vi "Export Dialog.vi"(8 "error in (no error)":errorcluster, 11 "Item Ref in":T1 format="%.0x") -> (0 "error out":errorcluster, 3 "Item Ref out":T1 format="%.0x")   [LabVIEW 2020, in "DSF System Explorer.lvlib"]
uses:
  DSF System Explorer.lvlib
  <vilib>/NI VeriStand/Custom Device API/Custom Device Item Ref.ctl
  Includes/DSF Core.lvlibp/Typedefs/DSF Engine Framework Configuration.ctl
  Includes/DSF Core.lvlibp/Typedefs/DSF Engine Plugin Configuration.ctl
  Includes/DSF Core.lvlibp/Typedefs/Core Plugin Configuration.ctl
  Includes/DSF Core.lvlibp/Typedefs/DSF Timing Info.ctl
  Includes/DSF Core.lvlibp/Typedefs/DSF Settings Info.ctl
  Includes/DSF Core.lvlibp/Typedefs/DSF Engine Plugin Thread Configuration.ctl
  Includes/DSF Core.lvlibp/Typedefs/Core Thread Configuration.ctl
  Includes/DSF Core.lvlibp/Typedefs/DSF Engine Transfer Group Configuration.ctl
  Includes/DSF Core.lvlibp/Typedefs/Core Group Configuration.ctl
  Includes/DSF Core.lvlibp/Typedefs/DSF Direction.ctl
  Includes/DSF Core.lvlibp/Typedefs/DSF Timeout Behavior.ctl
  Includes/DSF Core.lvlibp/Typedefs/DSF Engine Transfer Configuration.ctl
  Includes/DSF Core.lvlibp/Typedefs/Core Transfer Configuration.ctl
  Includes/DSF Core.lvlibp/Typedefs/DSF Engine Channel Configuration.ctl
  Includes/DSF Core.lvlibp/Typedefs/Core Channel Configuration.ctl
  Includes/DSF Core.lvlibp/Typedefs/DSF Data Type.ctl
  Includes/DSF Core.lvlibp
  Includes/DSF Core.lvlibp/Classes/Configuration/Core/Plugin/Plugin Configuration.lvclass
  Includes/DSF Core.lvlibp/Classes/Configuration/Core/Thread/Thread Configuration.lvclass
  Includes/DSF Core.lvlibp/Classes/Configuration/Core/Group/Group Configuration.lvclass
  Includes/DSF Core.lvlibp/Classes/Configuration/Core/Transfer/Transfer Configuration.lvclass
  Includes/DSF Core.lvlibp/Classes/Configuration/Core/Channel/Channel Configuration.lvclass
  Includes/DSF Core.lvlibp/Classes/Configuration Session/Configuration Session.lvclass
  Shared/DSF Shared.lvlib
  <vilib>/NI VeriStand/Custom Device API/Custom Device API.lvlib
panel:
  out "Duration":u32 format="%d ms"
  out "Version":string
  in  "Generate":bool
  in  "Save":bool
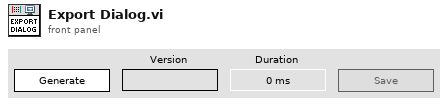
[diagram p1: front panel]
types:
  T1 = typedef "Custom Device API.lvlib/Custom Device Item Ref.ctl" = u64
  T2 = enum8{"Enabled", "Disabled", "Disabled and Grayed Out"}
  T3 = typedef "DSF Core.lvlibp/DSF Engine Framework Configuration.ctl" = cluster{"plugins":T4[]}
  T4 = typedef "DSF Core.lvlibp/DSF Engine Plugin Configuration.ctl" = cluster{"core":T5, "component settings":T7[], "threads":T8[]}
  T5 = typedef "DSF Core.lvlibp/Plugin Configuration.lvclass/Core Plugin Configuration.ctl" = cluster{"name":string, "components":string[], "cycle timing":T6}
  T6 = typedef "DSF Core.lvlibp/DSF Timing Info.ctl" = cluster{"priority":u64, "decimation":u64, "offset":u64}
  T7 = typedef "DSF Core.lvlibp/DSF Settings Info.ctl" = cluster{"component":string, "values":cluster{"key":string, "value":string}[]}
  T8 = typedef "DSF Core.lvlibp/DSF Engine Plugin Thread Configuration.ctl" = cluster{"core":T9, "component settings":T7[], "transfer groups":T10[]}
  T9 = typedef "DSF Core.lvlibp/Thread Configuration.lvclass/Core Thread Configuration.ctl" = cluster{"processor":i32, "priority offset":i16}
  T10 = typedef "DSF Core.lvlibp/DSF Engine Transfer Group Configuration.ctl" = cluster{"core":T11, "component settings":T7[], "transfers":T14[]}
  T11 = typedef "DSF Core.lvlibp/Group Configuration.lvclass/Core Group Configuration.ctl" = cluster{"name":string, "direction":T12, "cycle timing":T6, "timeout behavior":T13, "enable conversion":bool}
  T12 = typedef "DSF Core.lvlibp/DSF Direction.ctl" = enum8{"Tx", "Rx"}
  T13 = typedef "DSF Core.lvlibp/DSF Timeout Behavior.ctl" = enum8{"Increment Late Count", "Throw Error"}
  T14 = typedef "DSF Core.lvlibp/DSF Engine Transfer Configuration.ctl" = cluster{"core":T15, "component settings":T7[], "channels":T16[]}
  T15 = typedef "DSF Core.lvlibp/Transfer Configuration.lvclass/Core Transfer Configuration.ctl" = cluster{"name":string}
  T16 = typedef "DSF Core.lvlibp/DSF Engine Channel Configuration.ctl" = cluster{"core":T17, "component settings":T7[]}
  T17 = typedef "DSF Core.lvlibp/Channel Configuration.lvclass/Core Channel Configuration.ctl" = cluster{"name":string, "units":string, "engine data type":T18, "string data type":T18, "string offset":u64}
  T18 = typedef "DSF Core.lvlibp/DSF Data Type.ctl" = enum8{"Bool", "SGL", "DBL", "I8", "I16", "I32", "I64", "U8", "U16", "U32", "U64"}
  T19 = typedef "DSF Core.lvlibp/DSF Version Info.ctl" = cluster{"major":u32, "minor":u32, "fix":u32, "build":string}
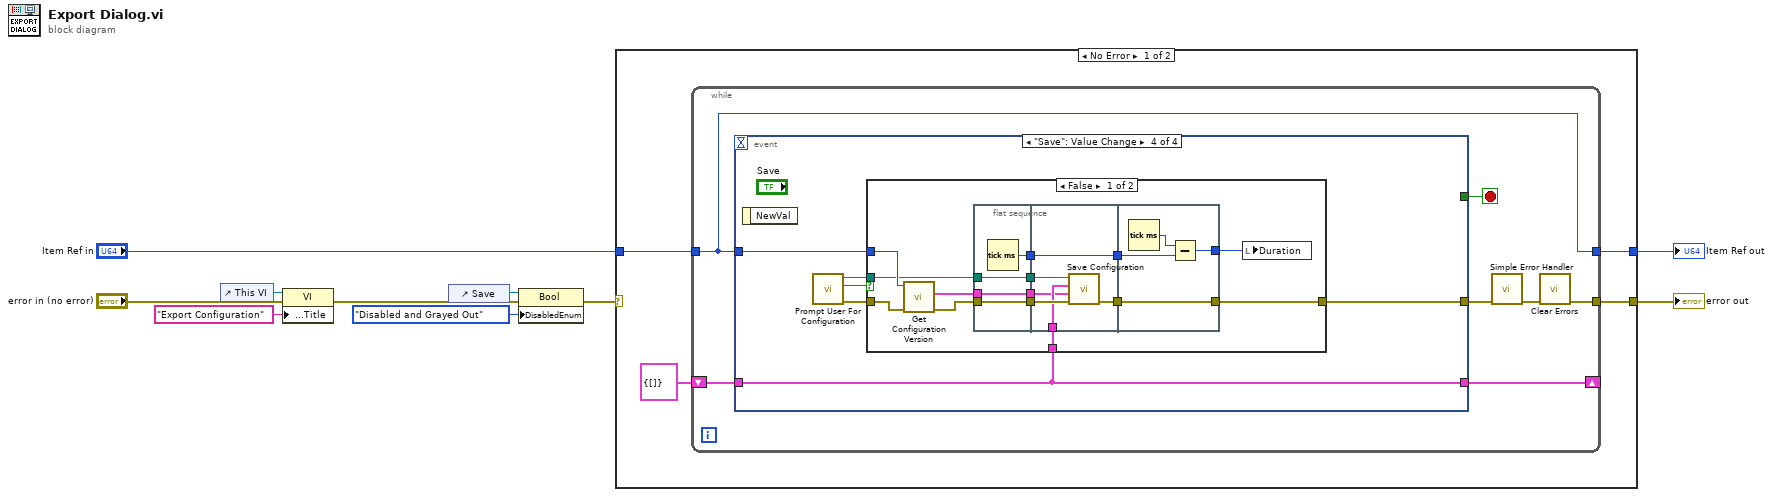
[diagram p0: block diagram]
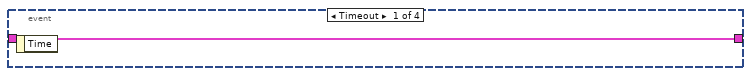
[diagram p2: hidden frame]
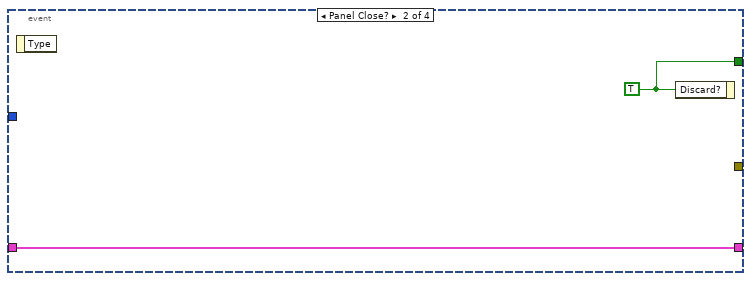
[diagram p3: hidden frame]
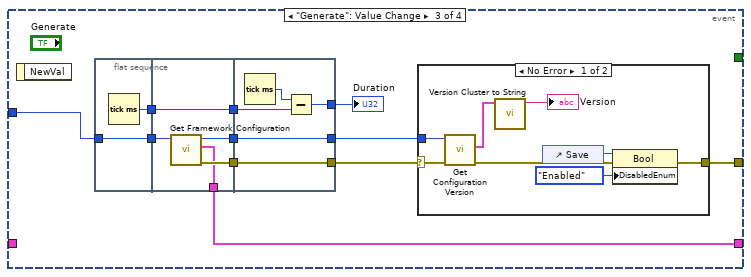
[diagram p4: hidden frame]
diagram:
  n1 = control-ref of="This VI"() -> (w7:refnum<vi>)
  n2 = property class="VI"(reference=w7, error in="error in (no error)", "Front Panel.Title"="Export Configuration" ("Front Panel Window:Title")) -> (error out=w2:errorcluster)  [unwired: 1 out]
  n3 = control-ref of="Save"() -> (w3:refnum<vi>)
  n4 = property class="Bool"(reference=w3, error in=w2, "DisabledEnum"=T2."Disabled and Grayed Out" ("Disabled")) -> (error out=w1:errorcluster)  [unwired: 1 out]
  n5 = case shown="No Error" w1 {
    selector: w1 -> [_ w92]
    tunnel: [w14 w92] -> w10
    tunnel: "Item Ref in" -> [w13 w93]
    tunnel: [w12 w93] -> w8
    frame No Error {
      n6 = while {
        tunnel: w13 -> [w15]
        tunnel: [w15] -> w12
        shift-right: [w17] -> _
        shift-left: T3 {"plugins"=[]} ("framework configuration") -> [w16]
        tunnel: [w20] -> w14
        stop <- w21 stop-if-true
        n7 = event shown="[3] \"Save\": Value Change" {
          selector: _ -> [_ _ _ _]
          dyn-events: _ -> [_ _ _ _]
          timeout: _ -> [_ _ _ _]
          tunnel: [_ w23 _ _] -> w21
          tunnel: [_ _ w30 w57] -> w19
          tunnel: w16 -> [w22 w24 _ w58]
          tunnel: [w22 w24 w29 w58] -> w17
          tunnel: w15 -> [_ _ w28 w59]
          event Timeout {
            n8 = event-data() -> ()  [unwired: 1 in, 1 out]
          }
          event Panel Close? {
            w23 = TRUE ("Discard?")
            n9 = event-data() -> ()  [unwired: 1 in, 1 out]
            n10 = event-data("Discard?"=w23) -> ()  [unwired: 1 in, 1 out]
          }
          event "Generate": Value Change {
            n11 = event-data() -> ()  [unwired: 1 in, 1 out]
            n12 = flat-sequence {
              tunnel: [w46] -> w35
              tunnel: w28 -> [w45]
              tunnel: [w45] -> w27
              tunnel: w35 -> [w51]
              tunnel: [w51] -> w34
              tunnel: [w50] -> w32
              tunnel: [w49] -> w29
              tunnel: w27 -> [w48]
              tunnel: [w47] -> w26
              tunnel: w34 -> [w56]
              tunnel: [w54] -> w33
              tunnel: w32 -> [w53]
              tunnel: [w53] -> w31
              tunnel: w26 -> [w52]
              tunnel: [w52] -> w25
              frame #0 {
                n13 = Tick Count (ms)() -> (millisecond timer value=w46:u32)
              }
              frame #1 {
                n14 = call "Get Framework Configuration.vi"("Item Ref in"=w48) -> ("error out"=w50:errorcluster, "framework configuration"=w49:T3, "Item Ref out"=w47:T1)  [unwired: 8 in]
              }
              frame #2 {
                n15 = Tick Count (ms)() -> (millisecond timer value=w55:u32)
                n16 = Subtract(x=w55, y=w56) -> (x-y=w54:u32)
              }
            }
            n17 = case shown="No Error" w31 {
              selector: w31 -> [w41 w44]
              tunnel: [w36 w44] -> w30
              tunnel: w25 -> [w40 _]
              frame No Error {
                n18 = call "Get Configuration Version.vi"("error in (no error)"=w41, "Item Ref in"=w40) -> ("error out"=w37:errorcluster, "version"=w38:T19)  [unwired: 7 in, 1 out]
                n19 = call "Version Cluster to String.vi"("version"=w38) -> ("version string"=→"Version":string)  [unwired: 9 in, 1 out]
                n20 = control-ref of="Save"() -> (w43:refnum<vi>)
                n21 = property class="Bool"(reference=w43, error in=w37, "DisabledEnum"=T2."Enabled" ("Disabled")) -> (error out=w36:errorcluster)  [unwired: 1 out]
              }
              frame Error {
              }
            }
            "Duration" <- w33
          }
          event "Save": Value Change {
            n22 = event-data() -> ()  [unwired: 1 in, 1 out]
            n23 = call "Prompt User For Configuration.vi"() -> ("error out"=w62:errorcluster, "cancelled"=w60:bool, "selected path"=w61:path)  [unwired: 9 in]
            n24 = case shown="False" w60 {
              tunnel: [w71 w91] -> w57
              tunnel: w62 -> [w69 w91]
              tunnel: w61 -> [w63 _]
              tunnel: w58 -> [w70 _]
              tunnel: w59 -> [w68 _]
              frame False {
                n25 = call "Get Configuration Version.vi"("error in (no error)"=w69, "Item Ref in"=w68) -> ("error out"=w67:errorcluster, "version"=w65:T19)  [unwired: 7 in, 1 out]
                n26 = flat-sequence {
                  tunnel: w67 -> [w80]
                  tunnel: [w80] -> w76
                  tunnel: [w79] -> w74
                  tunnel: w63 -> [w78]
                  tunnel: [w78] -> w66
                  tunnel: w65 -> [w77]
                  tunnel: [w77] -> w64
                  tunnel: w76 -> [w85]
                  tunnel: [w86] -> w75
                  tunnel: w74 -> [w84]
                  tunnel: [w84] -> w73
                  tunnel: w70 -> [w83]
                  tunnel: w66 -> [w82]
                  tunnel: w64 -> [w81]
                  tunnel: [w90] -> w71
                  tunnel: w75 -> [w90]
                  tunnel: w73 -> [w89]
                  tunnel: [w87] -> w72
                  frame #0 {
                    n27 = Tick Count (ms)() -> (millisecond timer value=w79:u32)
                  }
                  frame #1 {
                    n28 = call "Save Configuration.vi"("error in (no error)"=w85, "version (no change)"=w81, "framework configuration"=w83, "configuration file path"=w82) -> ("error out"=w86:errorcluster)  [unwired: 4 in, 3 out]
                  }
                  frame #2 {
                    n29 = Tick Count (ms)() -> (millisecond timer value=w88:u32)
                    n30 = Subtract(x=w88, y=w89) -> (x-y=w87:u32)
                  }
                }
                n31 = local write "Duration"(w72) -> ()
              }
              frame True {
              }
            }
          }
        }
        n32 = call <vilib>:"Simple Error Handler.vi"("error in (no error)"=w19) -> ("error out"=w18:errorcluster)  [unwired: 4 in, 4 out]
        n33 = call <vilib>:"Clear Errors.vi"("error in (no error)"=w18) -> ("error out"=w20:errorcluster)  [unwired: 5 in, 1 out]
      }
    }
    frame Error {
    }
  }
  "Item Ref out" <- w8
  "error out" <- w10
